vi "Initialize_DSC.vi"   [LabVIEW 2016]
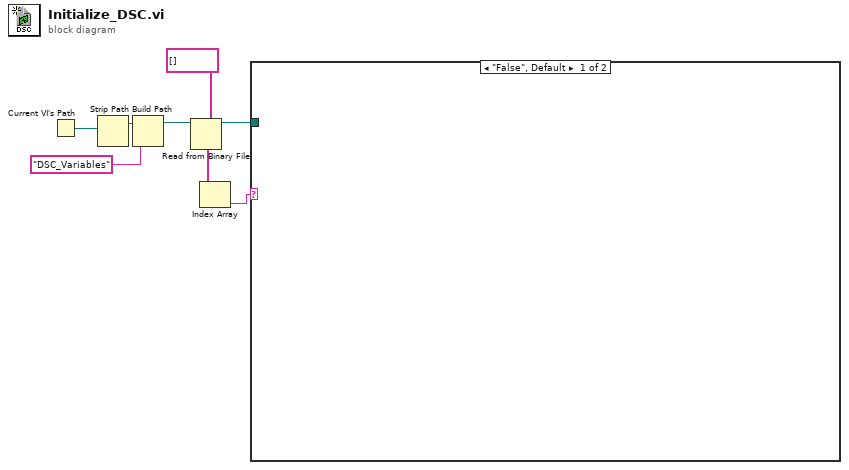
[diagram p0: block diagram]
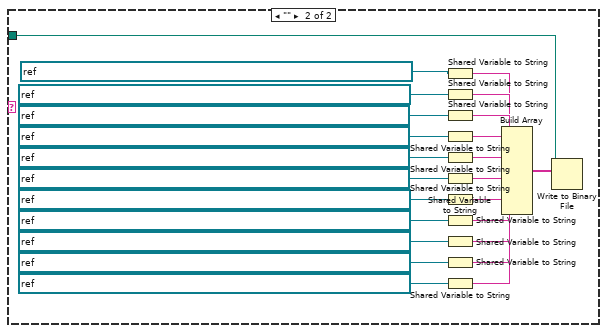
[diagram p2: hidden frame]
diagram:
  n1 = Current VI's Path() -> (path=w7:path)
  n2 = Strip Path(path=w7) -> (stripped path=w6:path)  [unwired: 1 out]
  n3 = Build Path(base path=w6, name or relative path="DSC_Variables") -> (appended path=w1:path)
  n4 = Read from Binary File(5:string[] [], 11:w1) -> (2:w3:string[])  [unwired: 4 in, 3 out]
  n5 = Index Array(array=w3) -> (element=w2:string)  [unwired: 1 in]
  n6 = case shown="\"False\", Default" w2 {
    tunnel: w1 -> [_ w8]
    frame "False", Default {
    }
    frame "" {
      n7 = Shared Variable to String(1:refnum<k21> "ni.var.psp://housesoftheholy/PPMS 1/PPMS 1 Magnetic Field" ("shared variable refnum in")) -> (0:w10:string)
      n8 = Shared Variable to String(1:refnum<k21> "ni.var.psp://housesoftheholy/PPMS 1/PPMS 1 Temperature" ("shared variable refnum in")) -> (0:w11:string)
      n9 = Shared Variable to String(1:refnum<k21> "ni.var.psp://housesoftheholy/PPMS 2/PPMS 2 Temperature" ("shared variable refnum in 3")) -> (0:w12:string)
      n10 = Shared Variable to String(1:refnum<k21> "ni.var.psp://housesoftheholy/PPMS 2/PPMS 2 Magnetic Field" ("shared variable refnum in 4")) -> (0:w13:string)
      n11 = Shared Variable to String(1:refnum<k21> "ni.var.psp://housesoftheholy/PPMS 2/PPMS 2 Helium Level" ("shared variable refnum in 5")) -> (0:w14:string)
      n12 = Shared Variable to String(1:refnum<k21> "ni.var.psp://housesoftheholy/Montana THZ 1/THZ 1 Temperature" ("shared variable refnum in 6")) -> (0:w15:string)
      n13 = Shared Variable to String(1:refnum<k21> "ni.var.psp://housesoftheholy/Cypher/Cypher Temperature" ("shared variable refnum in 9")) -> (0:w16:string)
      n14 = Shared Variable to String(1:refnum<k21> "ni.var.psp://housesoftheholy/MNK_18T/MNK_TC_T3" ("shared variable refnum in 10")) -> (0:w17:string)
      n15 = Shared Variable to String(1:refnum<k21> "ni.var.psp://housesoftheholy/MFP3D/MFP3D Temperature" ("shared variable refnum in 11")) -> (0:w18:string)
      n16 = Shared Variable to String(1:refnum<k21> "ni.var.psp://housesoftheholy/PPMSDR/PPMSDR Magnetic Field (Oe)" ("shared variable refnum in 12")) -> (0:w19:string)
      n17 = Shared Variable to String(1:refnum<k21> "ni.var.psp://housesoftheholy/PPMSDR/PPMSDR Temperature (K)" ("shared variable refnum in 13")) -> (0:w20:string)
      n18 = Build Array(w10, w11, w12, w13, w14, w15, w16, w17, w18, w19, w20) -> (w9:string[])
      n19 = Write to Binary File(file (use dialog)=w8, data=w9) -> ()  [unwired: 4 in, 3 out]
    }
  }
